vi "ReadInitialAverages.vi"() -> (2 "avgOut":bool[][](array[boolean]))   [LabVIEW 2016]
panel:
  out "intMatrix4x8":i32[][](array[numeric])
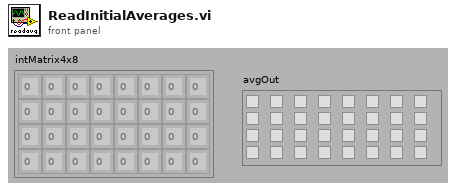
[diagram p1: front panel]
types:
  T1 = enum16{"open", "replace", "create", "open or create", "replace or create", "replace or create with confirmation"}
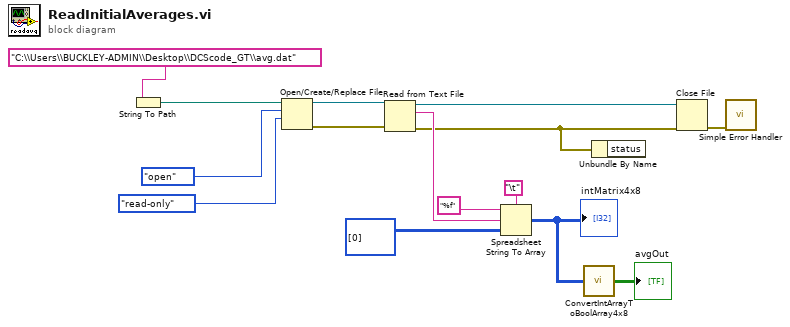
[diagram p0: block diagram]
diagram:
  n1 = String To Path(string="C:\\Users\\BUCKLEY-ADMIN\\Desktop\\DCScode_GT\\avg.dat") -> (path=w8:path)
  n2 = Open/Create/Replace File(file path (use dialog)=w8, operation (0:open)=T1."open", access (0:read/write)=enum16{"read/write", "read-only", "write-only"}."read-only") -> (refnum out=w7:refnum<file>, error out=w6:errorcluster)  [unwired: 1 in, 3 out]
  n3 = Read from Text File(file (use dialog)=w7, error in=w6) -> (refnum out=w4:refnum<file>, text=w13:string, error out=w3:errorcluster)  [unwired: 3 out]
  n4 = Spreadsheet String To Array(delimiter (Tab)="\t", format string="%f", spreadsheet string=w13, array type (2D Dbl)=i32[][] [[0]]) -> (array=w1:i32[][])
  "intMatrix4x8" <- w1
  n5 = call "ConvertIntArrayToBoolArray4x8.vi"("intMatrix4x8"=w1) -> ("avgOut"=→"avgOut":bool[][])  [unwired: 14 out]
  n6 = Unbundle By Name(w3) -> ()  [unwired: 1 out]
  n7 = Close File(refnum=w4, error in=w3) -> (error out=w5:errorcluster)  [unwired: 1 out]
  n8 = call <vilib>:"Simple Error Handler.vi"("error in (no error)"=w5) -> ()  [unwired: 1 in, 8 out]
